vi "NBFM.vi"() -> ()   [LabVIEW 2013]
uses:
  <vilib>/addons/Modulation/Analog/MT Passband PLL.vi
  <vilib>/sound2/lvsound2.llb/Sound File Info (path).vi
  <vilib>/sound2/lvsound2.llb/Sound File Read Open.vi
  <vilib>/sound2/lvsound2.llb/Sound File Read (DBL).vi
  <vilib>/Waveform/WDTOps.llb/WDT Get Waveform Subset DBL.vi
  <vilib>/express/express analysis/Spectral/Block/exnSpectralBlock spectral measurements RMS poly.vi
  <vilib>/express/express analysis/Spectral/Block/exnSpectralBlock spectral measurements RMS DDT.vi
  <vilib>/express/express analysis/Spectral/XNode/ExpressSpectralMeasurementsBlockNode.xnode
  <vilib>/addons/Modulation/niAMT.lvlib
panel:
  out "Estimated Freq.":dbl=100000.0 caption="Frequency"
  in  "Modulated Signal Source":enum32{"Single Tone", "From File"}(tab)
  in  "ST Frequency":dbl=2000.0 caption="Frequency"
  in  "ST Amplitude":dbl=1.0 caption="Amplitude"
  in  "Resample Rate":dbl=1000000.0 format="%#_6f"
  in  "Duration":dbl=44100.0
  in  "WAV Path":path=path "E:/07/0409/mozart.wav" caption="Path"
  in  "Normalized Peak Amplitude":dbl=1.0 caption="Peak Amplitude"
  in  "WAV Sample Rate":dbl=44100.0 caption="dt"
  in  "LPF Cut-Off":dbl=5000.0 caption="Lower Cut-Off"
  in  "SNR (dB)":dbl(slide)=30.0 caption="Standard deviation" scale=-20.0..50.0
  out "Recovered Signal":dynamicdata(graph)
  out "Baseband":dynamicdata(graph)
  out "FM FFT":dynamicdata(graph)
  out "FM Wave":dynamicdata(graph)
  in  "Carrier Amp.":dbl=1.0 caption="Amplitude"
  in  "stop":bool
  in  "k_f":dbl(slide)=400.0 scale=0.0..1000.0
  in  "Carrier Freq.":dbl=100000.0 caption="Frequency"
  # "Frequency Modulation"
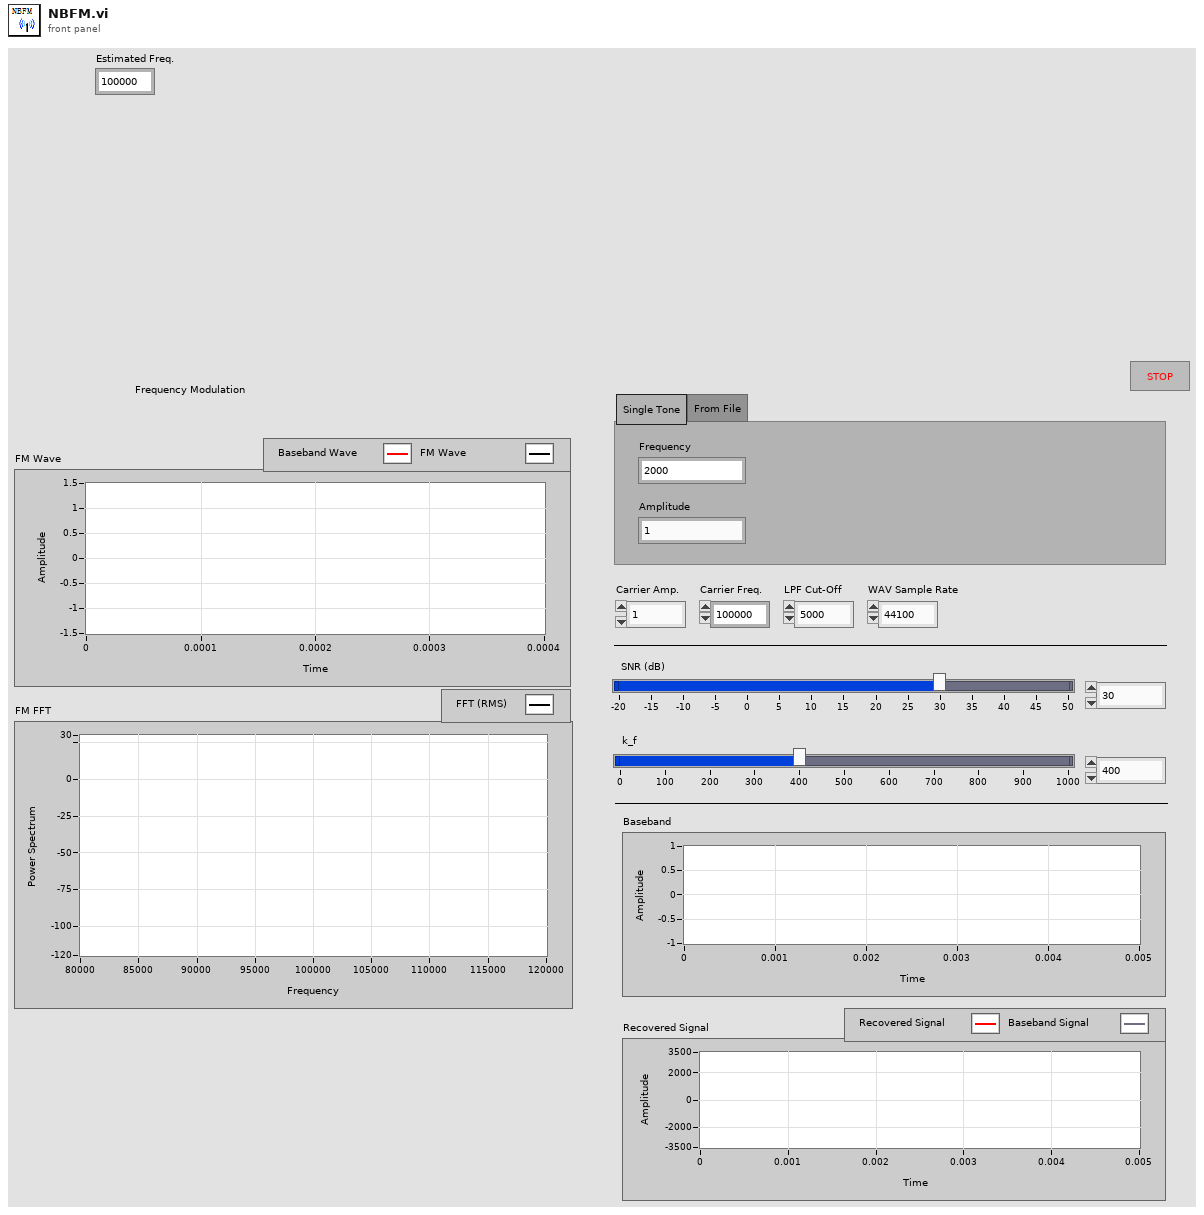
[diagram p1: front panel]
types:
  T1 = cluster{"averaging mode":u16, "weighting mode":u16, "number of averages":u32}
  T2 = cluster{"dB On (F)":bool, "unwrap phase (F)":bool, "convert to degree (F)":bool}
  T3 = typedef "Sound File Refnum.ctl" = refnum<file>
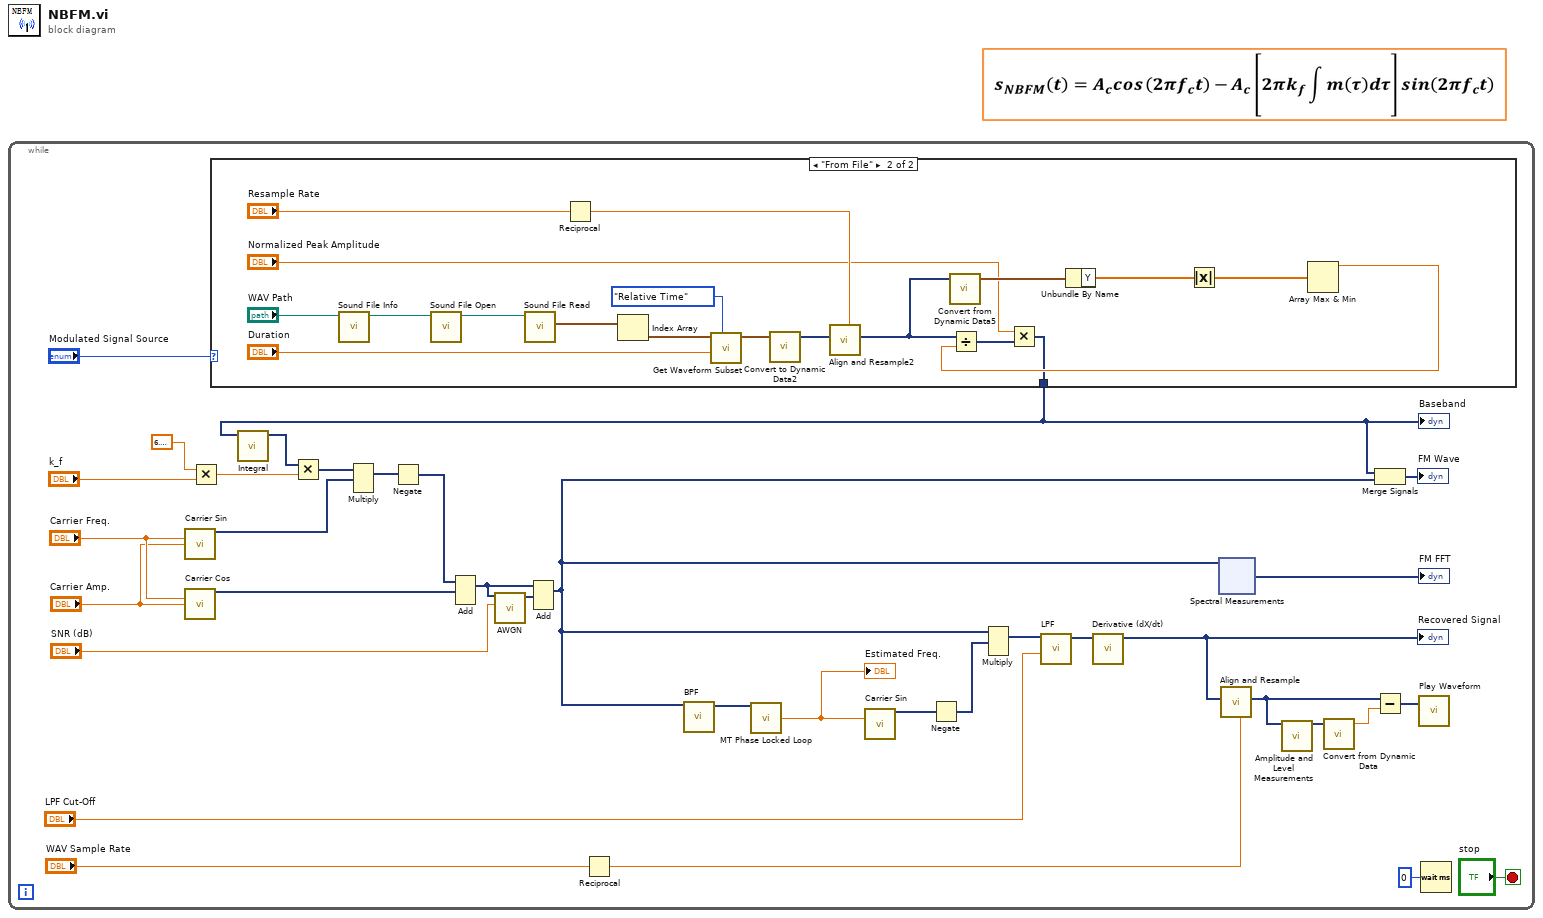
[diagram p0: block diagram]
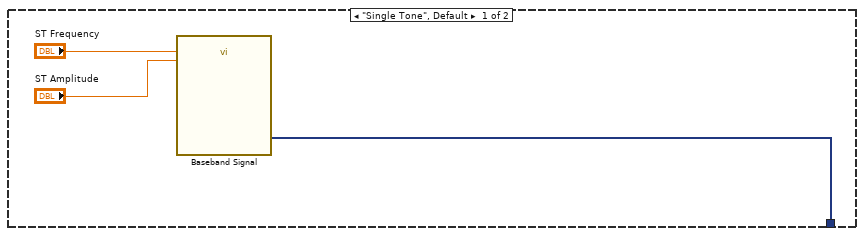
[diagram p2: hidden frame]
diagram:
  n1 = while {
    stop <- "stop" stop-if-true
    n2 = call "Carrier Sin"("Frequency"="Carrier Freq.", "Amplitude"="Carrier Amp.") -> ("Sine"=w20:dynamicdata)  [unwired: 12 in, 1 out]
    n3 = call "Carrier Cos"("Frequency"="Carrier Freq.", "Amplitude"="Carrier Amp.") -> ("Sine"=w13:dynamicdata)  [unwired: 12 in, 1 out]
    n4 = Multiply(x=6.283185307179586, y="k_f") -> (x*y=w14:dbl)
    n5 = case shown="\"From File\"" "Modulated Signal Source" {
      tunnel: [w36 w40] -> w15
      frame "Single Tone", Default {
        n6 = call "Baseband Signal"("Frequency"="ST Frequency", "Amplitude"="ST Amplitude") -> ("Sine"=w36:dynamicdata)  [unwired: 12 in, 1 out]
      }
      frame "From File" {
        n7 = call-poly <vilib>:"Sound File Info.vi"("path"="WAV Path") -> ("path out"=w55:path)  [unwired: 7 in, 3 out]
        n8 = call-poly <vilib>:"Sound File Open.vi"("path"=w55) -> ("sound file refnum"=w57:T3)  [unwired: 9 in, 1 out]
        n9 = call-poly <vilib>:"Sound File Read.vi"("sound file refnum"=w57) -> ("data"=w52:waveform(dbl)[])  [unwired: 6 in, 4 out]
        n10 = Reciprocal(x="Resample Rate") -> (1/x=w48:dbl)
        n11 = Index Array(array=w52) -> (element=w53:waveform(dbl))  [unwired: 1 in]
        n12 = call-poly <vilib>:"Get Waveform Subset.vi"("start/duration format"=enum16{"Relative Time"}."Relative Time", "duration"="Duration", "waveform in"=w53) -> ("waveform out"=w47:waveform(dbl))  [unwired: 3 in, 3 out]
        n13 = call "Convert to Dynamic Data2"("Waveform"=w47) -> ("Dynamic Data Type"=w42:dynamicdata)  [unwired: 3 in]
        n14 = call "Align and Resample2"("dt"=w48, "Signals"=w42) -> ("Resampled Signals"=w43:dynamicdata)  [unwired: 7 in, 2 out]
        n15 = call "Convert from Dynamic Data5"("Dynamic Data Type"=w43) -> ("Waveform"=w50:waveform(dbl))  [unwired: 3 in]
        n16 = Unbundle By Name(w50) -> ("Y"=w44:dbl[])
        n17 = Absolute Value(x=w44) -> (abs(x)=w46:dbl[])
        n18 = Array Max & Min(array=w46) -> (max value=w45:dbl)  [unwired: 3 out]
        n19 = Divide(x=w43, y=w45) -> (x/y=w41:dynamicdata)
        n20 = Multiply(x="Normalized Peak Amplitude", y=w41) -> (x*y=w40:dynamicdata)
      }
    }
    "Baseband" <- w15
    n21 = call "Integral"("Signals"=w15) -> ("Result"=w16:dynamicdata)  [unwired: 5 in, 1 out]
    n22 = Multiply(x=w16, y=w14) -> (x*y=w12:dynamicdata)
    n23 = Multiply(1:w20, 2:w12) -> (0:w11:dynamicdata)  [unwired: 1 in, 1 out]
    n24 = Negate(x=w11) -> (-x=w10:dynamicdata)
    n25 = Add(1:w13, 2:w10) -> (0:w21:dynamicdata)  [unwired: 1 in, 1 out]
    n26 = call "AWGN.vi"("SNR (dB)"="SNR (dB)", "Dynamic Data"=w21) -> ("DC with Gaussian Noise"=w25:dynamicdata)  [unwired: 9 in]
    n27 = Add(1:w25, 2:w21) -> (0:w4:dynamicdata)  [unwired: 1 in, 1 out]
    n28 = Reciprocal(x="WAV Sample Rate") -> (1/x=w22:dbl)
    n29 = call "BPF"("Signal"=w4) -> ("Filtered Signal"=w5:dynamicdata)  [unwired: 9 in, 1 out]
    n30 = call-poly <vilib>:"MT Phase Locked Loop.vi"("passband waveform"=w5) -> ("estimated carrier frequency (Hz)"=w8:dbl)  [unwired: 10 in, 4 out]
    "Estimated Freq." <- w8
    n31 = call "Carrier Sin"("Frequency"=w8) -> ("Sine"=w9:dynamicdata)  [unwired: 13 in, 1 out]
    n32 = Negate(x=w9) -> (-x=w6:dynamicdata)
    n33 = Multiply(1:w6, 2:w4) -> (0:w7:dynamicdata)  [unwired: 1 in, 1 out]
    n34 = call "LPF"("Lower Cut-Off"="LPF Cut-Off", "Signal"=w7) -> ("Filtered Signal"=w2:dynamicdata)  [unwired: 8 in, 1 out]
    n35 = call "Derivative (dX/dt)"("Signals"=w2) -> ("Result"=w1:dynamicdata)  [unwired: 5 in, 1 out]
    "Recovered Signal" <- w1
    n36 = xnode ("Spectral Measurements")("Signals"=w4) -> ("FFT - (RMS)"=→"FM FFT":dynamicdata)  [unwired: 1 in, 2 out]
    n37 = call "Align and Resample"("dt"=w22, "Signals"=w1) -> ("Resampled Signals"=w18:dynamicdata)  [unwired: 7 in, 2 out]
    n38 = call "Amplitude and Level Measurements"("Signals"=w18) -> ("Mean (DC)"=w31:dynamicdata)  [unwired: 13 in, 1 out]
    n39 = call "Convert from Dynamic Data"("Dynamic Data Type"=w31) -> ("Scalar"=w32:dbl)  [unwired: 3 in]
    n40 = Merge Signals(w15, w4) -> (→"FM Wave":dynamicdata)
    n41 = Subtract(x=w18, y=w32) -> (x-y=w19:dynamicdata)
    n42 = call "Play Waveform"("Data"=w19) -> ()  [unwired: 18 in, 1 out]
    n43 = Wait (ms)(milliseconds to wait=u32 0) -> ()  [unwired: 1 out]
  }
